vi "DAQ 1SDI v00.vi"() -> ()   [LabVIEW 2013]
uses:
  <instrlib>/niScope/Controls/niScope vertical coupling.ctl
  Strict Type Defs/type_meas_enum.ctl
  Strict Type Defs/Monitor switches.ctl
  Global VIs/shotnoise.vi
panel:
  in  "Monitors":enum32{"Monitors On", "Monitors Off"}(tab)
  out "Variance 1 normalised to SNL":dbl(graph)=-0.09698706546327589
  out "Conditional variance":dbl(graph)=0.9777105612597436
  out "Variance 2 normalised to SNL":dbl(graph)=0.43220629575348973
  out "covariance":dbl(graph)=0.015043042666783312
  out "Signal 2":dbl[](graph)
  out "Signal 1":dbl[](graph)
  out "Loop count":i32=2500
  in  "stop":bool
  in  "Settings":enum32{"Settings and Record", "Under the hood"}(tab)
  out "Video bandwidth (Hz)":dbl=3333.3333333333335
  in  "Minimum sample rate (S/s)":dbl=100000000.0 format="%#_6p"
  in  "Reference position":dbl(slide)=50.0 scale=0.0..100.0
  in  "max time (s)":dbl=10.0 caption="Time to run (s)"
  in  "Channel parameters":T2(array[cluster])=[{"Channel name"="0", "Input impedance (Ohms)"=2, "Maximum input frequency (Hz)"=30000000.0, "vertical coupling"=1, "Probe attenuation"=1.0, "Vertical range (V)"=0.2, "Vertical offset"=0.0, "channel enabled"=TRUE}, {"Channel name"="1", "Input impedance (Ohms)"=2, "Maximum input frequency (Hz)"=30000000.0, "vertical coupling"=1, "Probe attenuation"=1.0, "Vertical range (V)"=0.2, "Vertical offset"=0.0, "channel enabled"=TRUE}] {"Input impedance (Ohms)" items=["1 mega ohm"=0, "50 ohms"=2]; "Maximum input frequency (Hz)" format="%#_6p"; "vertical coupling" items=["AC", "DC", "Ground"]}
  in  "IIR filter specifications":T3={"Topology"=enum."Butterworth", "Type"=enum."Bandpass", "Order"=6, "Lower Fc"=2700000.0, "Upper Fc"=3100000.0, "PB Ripple"=1.0, "SB Attenuation"=60.0} {"PB Ripple" format="%0.2f"; "SB Attenuation" format="%0.2f"; "Lower Fc" format="%0.2p"; "Upper Fc" format="%0.2p"}
  in  "File location":path=path "C:/ni-rt/LabVIEW Data/June4"
  in  "Record Data":bool
  in  "Type of measurement":T4
  in  "File root name":string="testJune"
  in  "Number of samples 2":i32=30000 format="%.0p"
  in  "reset sn":bool
  in  "Shot noise start":bool
  out "error out":errorcluster caption="error out final"
  out "Actual samples acquired ch 0":i32=30000
  out "Actual samples acquired ch 1":i32=30000
  out "SN loop count":i64=44
  out "SN":dbl[](array[numeric])=[0.0011925520800490743, 8.097186254673786e-06]
  out "Parameters values file":string="PARAMETERS VALUES\r\rTuesday, September 12, 2006\r1:42 AM\r\rMaster ch 0 <-> HD1 AC a-b\nMaster ch 1 <-> HD2 AC a-b\n\r\r\r\rSample rate : \rMaster : 100.000000E+6 Samples per second\rNumber of samples :\rMaster ch 0 : 30.000000E+3\rMaster ch 1 : 30.000000E+3\rFiles names : \rtestJune_sqz_ParametersValues_30000.txt\rtestJune_sqz_mch0_30000.txt\rtestJune_sqz_mch1_30000.txt\rtestJune_sqz_mch01_60000.txt\r"
  in  "DAQ Card":refnum<k15>="PXI1Slot7"
  in  "Monitor Switches":T5
  # "Variance won't be displayed until shot noise is taken"
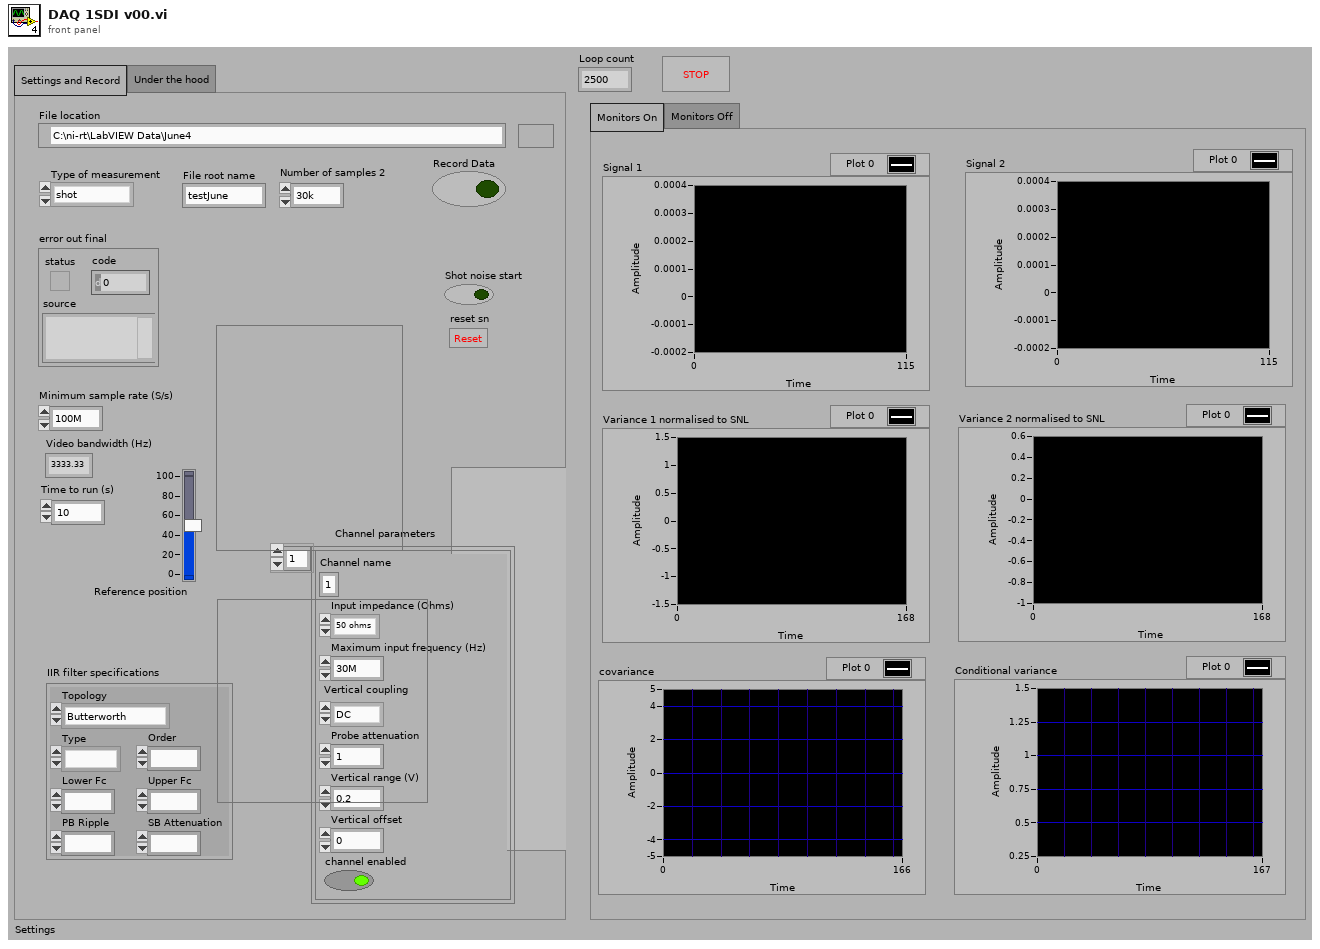
[diagram p1: front panel]
types:
  T1 = typedef "niScope vertical coupling.ctl" = i32
  T2 = cluster{"Channel name":string, "Input impedance (Ohms)":u32, "Maximum input frequency (Hz)":dbl, "vertical coupling":T1, "Probe attenuation":dbl, "Vertical range (V)":dbl, "Vertical offset":dbl, "channel enabled":bool}[]
  T3 = cluster{"Topology":enum16{"Off", "Butterworth", "Chebyshev", "Inverse Chebyshev", "Elliptic", "Bessel"}, "Type":enum16{"Lowpass", "Highpass", "Bandpass", "Bandstop"}, "Order":i32, "Lower Fc":dbl, "Upper Fc":dbl, "PB Ripple":dbl, "SB Attenuation":dbl}
  T4 = typedef "type_meas_enum.ctl" = enum16{"shot", "x", "p", "electronic"}
  T5 = typedef "Monitor switches.ctl" = cluster{"Signal 1 On":bool, "Signal 2 On":bool, "Variance 1 On":bool, "Variance 2 On":bool, "Cov On":bool, "Cond. On":bool, "Monitors On":bool}
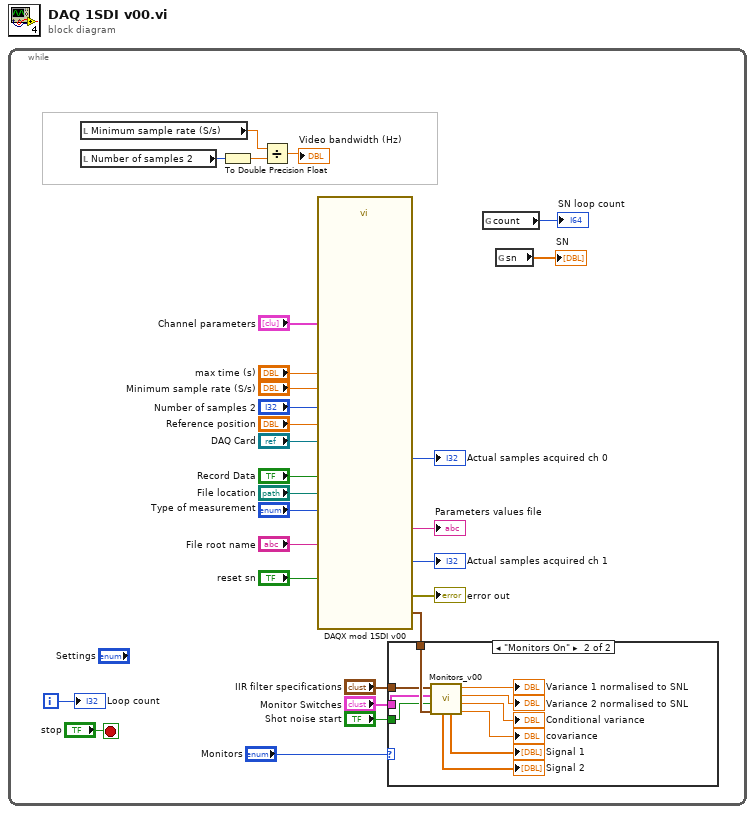
[diagram p0: block diagram]
diagram:
  n1 = while {
    i -> [w10]
    stop <- "stop" stop-if-true
    n2 = local read "Minimum sample rate (S/s)"() -> (w26:dbl)
    n3 = local read "Number of samples 2"() -> (w28:i32)
    n4 = To Double Precision Float(number=w28) -> (double precision float=w25:dbl)
    n5 = Divide(x=w26, y=w25) -> (x/y=→"Video bandwidth (Hz)":dbl)
    n6 = call "DAQX mod 1SDI v00.vi"("resource name"="DAQ Card", "Record Data"="Record Data", "numSamples"="Number of samples 2", "max time (s)"="max time (s)", "min sample rate"="Minimum sample rate (S/s)", "File location"="File location", "reference position"="Reference position", "Type of\nmeasurement"="Type of measurement", "Name root"="File root name", "channel parameters"="Channel parameters", "reset sn"="reset sn") -> ("wfm out"=w6:waveform(dbl)[], "Parameters values file"=→"Parameters values file":string, "actualSamples 0"=→"Actual samples acquired ch 0":i32, "actualSamples 1"=→"Actual samples acquired ch 1":i32, "error out"=→"error out":errorcluster)  [unwired: 5 in, 7 out]
    n7 = case shown="\"Monitors On\"" "Monitors" {
      tunnel: w6 -> [_ w38]
      tunnel: "IIR filter specifications" -> [_ w31]
      tunnel: "Monitor Switches" -> [_ w30]
      tunnel: "Shot noise start" -> [_ w29]
      frame "Monitors Off" {
      }
      frame "Monitors On" {
        n8 = call "Monitors_v00.vi"("wfm"=w38, "Shot noise start"=w29, "Monitor Switches"=w30, "IIR filter specifications"=w31) -> ("covariance"=→"covariance":dbl, "conditional variance"=→"Conditional variance":dbl, "Variance 2 normalised to SNL"=→"Variance 2 normalised to SNL":dbl, "Variance 1 normalised to SNL"=→"Variance 1 normalised to SNL":dbl, "Signal 1"=→"Signal 1":dbl[], "Signal 2"=→"Signal 2":dbl[])  [unwired: 2 in]
      }
    }
    n9 = global read "shotnoise.vi" "count"() -> (→"SN loop count":i64)
    n10 = global read "shotnoise.vi" "sn"() -> (→"SN":dbl[])
    "Loop count" <- w10
  }
